vi "Read Props.vi"(8 "error in (no error)":errorcluster, 11 "DblControlEditorPanel in":refnum<class "DblControlEditorPanel.lvclass">) -> (0 "error out":errorcluster, 2 "Props":T1)   [LabVIEW 2020, in "VolatusGUIControls.lvlib" / "DblControlEditorPanel.lvclass"]
uses:
  DblControlEditorPanel.lvclass
  Props.ctl
  JSON Props.ctl
  DblControlEditorPanel.lvclass/DblControlEditorPanel.ctl
  dd1baaf3-e1aa-4c54-b388-d9d93c741139.vi
  <vilib>/JDP Science/JSONtext/JSON text to Variant.vi
  <vilib>/JDP Science/JSONtext/LVClass Serializer/JSONtext LVClass Serializer.lvclass
  VolatusGUIControls.lvlib
  VolatusGUIEditorCore/Numeric Text Props.ctl
  VolatusGUIEditorCore/VolatusGUIEditorCore.lvlib
  VolatusGUIEditorCore/Position Props.ctl
  VolatusGUIEditorCore/Label Props.ctl
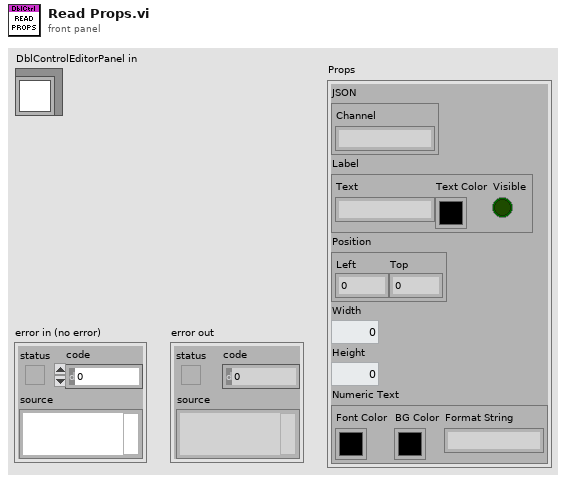
[diagram p1: front panel]
types:
  T1 = typedef "VolatusGUIControls.lvlib/DblControlEditorPanel.lvclass/Props.ctl" = cluster{"JSON":T2, "Label":T3, "Position":T4, "Width":u16, "Height":u16, "Numeric Text":T5}
  T2 = typedef "VolatusGUIControls.lvlib/DblControlEditorPanel.lvclass/JSON Props.ctl" = cluster{"Channel":string}
  T3 = typedef "VolatusGUIEditorCore.lvlib/Label Props.ctl" = cluster{"Text":string, "Text Color":u32, "Visible":bool}
  T4 = typedef "VolatusGUIEditorCore.lvlib/Position Props.ctl" = cluster{"Left":i32, "Top":i32}
  T5 = typedef "VolatusGUIEditorCore.lvlib/Numeric Text Props.ctl" = cluster{"Font Color":u32, "BG Color":u32, "Format String":string}
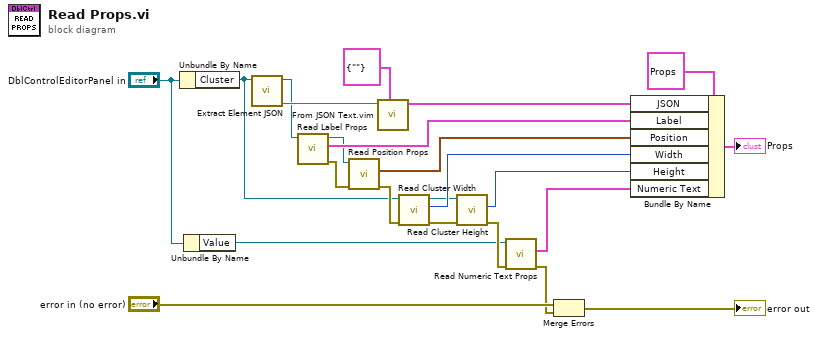
[diagram p0: block diagram]
diagram:
  n1 = Unbundle By Name("DblControlEditorPanel in") -> ("Cluster"=w9:refnum<vi>)
  n2 = Unbundle By Name("DblControlEditorPanel in") -> ("Value"=w14:refnum<vi>)
  n3 = call "Extract Element JSON.vi"("Ctl Refnum in"=w9) -> ("JSON"=w20:string, "Ctl Refnum"=w10:refnum<vi>)  [unwired: 7 in, 2 out]
  n4 = call "Read Label Props.vi"("Ctl Refnum in"=w10) -> ("error out"=w8:errorcluster, "Label Props"=w13:T3, "Ctl Refnum"=w12:refnum<vi>)  [unwired: 8 in]
  n5 = call "Read Position Props.vi"("error in (no error)"=w8, "Ctl Refnum in"=w12) -> ("error out"=w22:errorcluster, "Position Props"=w11:T4)  [unwired: 7 in, 1 out]
  n6 = call "From JSON Text.vim"("Data Type and Default Value"=T2 {"Channel"=""} ("JSON Props"), "JSON"=w20) -> ("Data out"=w16:T2)  [unwired: 8 in, 1 out]
  n7 = call "Read Cluster Width.vi"("error in (no error)"=w22, "Cluster in"=w9) -> ("error out"=w5:errorcluster, "Width"=w7:i32, "Cluster"=w6:refnum<vi>)  [unwired: 7 in]
  n8 = call "Read Cluster Height.vi"("error in (no error)"=w5, "Cluster in"=w6) -> ("error out"=w23:errorcluster, "Height"=w4:i32)  [unwired: 7 in, 1 out]
  n9 = call "Read Numeric Text Props.vi"("error in"=w23, "Control in"=w14) -> ("error out"=w1:errorcluster, "Numeric Text Props"=w3:T5)  [unwired: 7 in, 1 out]
  n10 = Merge Errors("error in (no error)", w1) -> (→"error out":errorcluster)
  n11 = Bundle By Name(cluster=T1 {"JSON"={"Channel"=""}, "Label"={"Text"="", "Text Color"=0, "Visible"=FALSE}, "Position"={"Left"=0, "Top"=0}, "Width"=0, "Height"=0, "Numeric Text"={"Font Color"=0, "BG Color"=0, "Format String"=""}} ("Props"), "JSON"=w16, "Label"=w13, "Position"=w11, "Width"=w7, "Height"=w4, "Numeric Text"=w3) -> (→"Props":T1)
